vi "Write conditional terminal.vi"(5 "conditional terminal":refnum<class "Terminal.lvclass">, 9 "LoopTunnel in":refnum<class "LoopTunnel.lvclass">) -> (3 "LoopTunnel out":refnum<class "LoopTunnel.lvclass">)   [LabVIEW 2014, in "LoopTunnel.lvclass"]
uses:
  LoopTunnel.lvclass
  Terminal/Terminal.lvclass
  LoopTunnel.lvclass/LoopTunnel.ctl
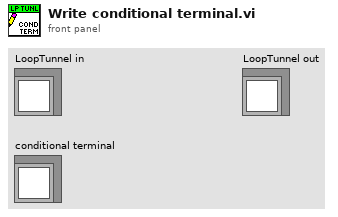
[diagram p1: front panel]
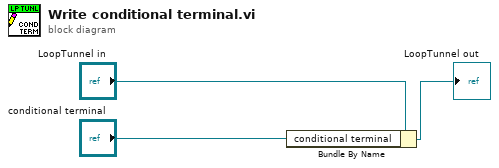
[diagram p0: block diagram]
diagram:
  n1 = Bundle By Name(cluster="LoopTunnel in", "conditional terminal"="conditional terminal") -> (→"LoopTunnel out":refnum<class "LoopTunnel.lvclass">)
